vi "Create Combination 2.vi"(6 "Element In":i32, 7 "Combinations In":dbl[][](array[numeric]), 9 "Array":dbl[](array[numeric])=[1.0, 2.0, 3.0, 4.0, 5.0], 10 "Index":i32, 11 "Temp Combination":dbl[](array[numeric])) -> (4 "Element Out":i32, 5 "Combinations Out":dbl[][](array[numeric]))   [LabVIEW 2018]
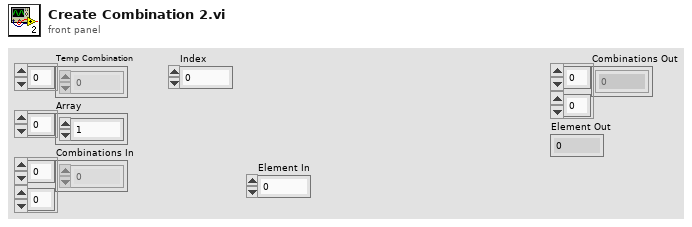
[diagram p1: front panel]
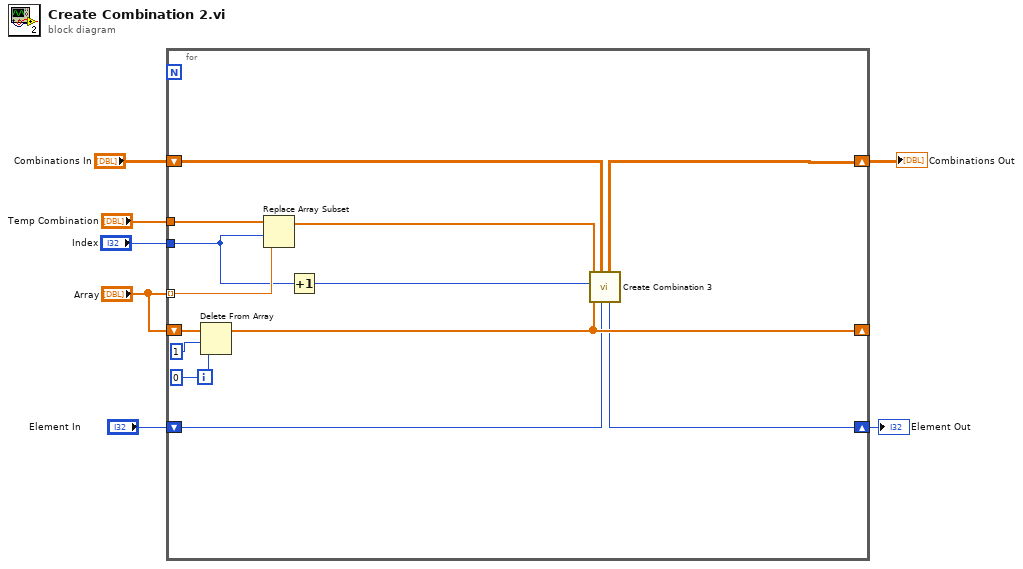
[diagram p0: block diagram]
diagram:
  n1 = for {
    tunnel: "Temp Combination" -> [w19]
    tunnel: "Array" -> [w18] mode=indexing
    shift-right: [w13] -> _
    shift-left: "Array" -> [w20]
    tunnel: "Index" -> [w15]
    shift-right: [w11] -> w4
    shift-left: "Combinations In" -> [w12]
    shift-right: [w8] -> w1
    shift-left: "Element In" -> [w9]
    n2 = Delete From Array(array=w20, length=1, index=0) -> (array with subset deleted=w13:dbl[])  [unwired: 1 out]
    n3 = Replace Array Subset(array=w19, new element=w18, index=w15) -> (w14:dbl[])
    n4 = Increment(x=w15) -> (x+1=w10:i32)
    n5 = call "Create Combination 3.vi"("Element"=w9, "Combinations In"=w12, "Array"=w13, "Index"=w10, "Temp Combination"=w14) -> ("Element out"=w8:i32, "Combinations Out"=w11:dbl[][])  [unwired: 5 in]
  }
  "Combinations Out" <- w4
  "Element Out" <- w1
